vi "Set - Wash Sequence.vi"(8 "error in (no error)":errorcluster, 10 "Wash Sequence":T1[](array[typedef]), 11 "View Model":T2) -> (0 "error out":errorcluster, 3 "View Model":T2)   [LabVIEW 2017]
doc: "Set actual value of Wash Sequence to DVR."
uses:
  Controls/View Model.ctl
  Controls/Shared Model.ctl
  Error Handler/Controls/Error Model.ctl
  Error Handler/Controls/Error Data.ctl
  Error Handler/Controls/Error Level.ctl
  Configuration/Controls/Config Model.ctl
  Configuration/Controls/Config Record.ctl
  Configuration/Controls/Config Data.ctl
  Configuration/Controls/Config Command.ctl
  Controller/Controls/Controler Model.ctl
  Views/Vehicle Position View/Controls/Vehicle - Station Slider.ctl
  Controller/Controls/Controller - Wash Step.ctl
  Views/Entry Console View/Controls/Entry Console - Wash Steps.ctl
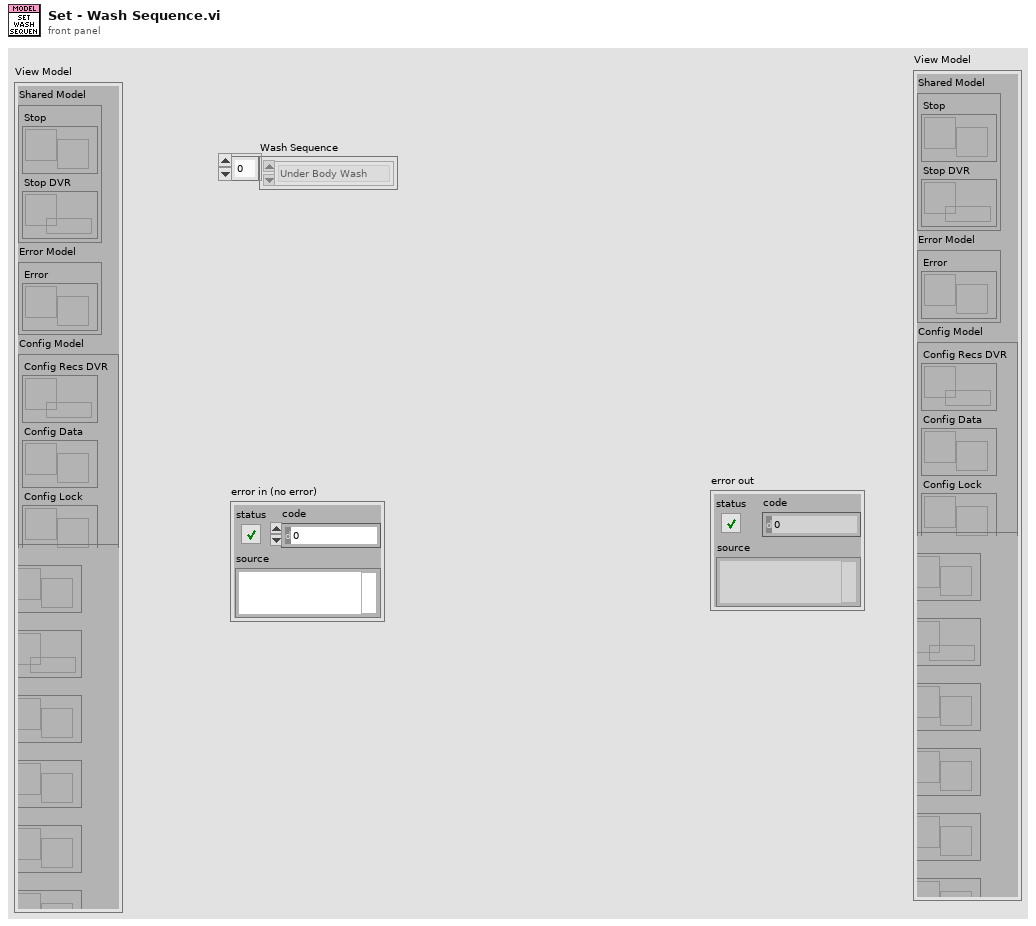
[diagram p1: front panel]
types:
  T1 = typedef "Controller - Wash Step.ctl" = enum16{"Under Body Wash", "Bug Remover", "Pre-Soak", "High Pressure Wash", "Low Pressure Wax", "Spot Free Rinse", "Tire Shine Foam", "Air Dry"}
  T2 = typedef "View Model.ctl" = cluster{"Shared Model":T3, "Error Model":T4, "Config Model":T5, "Controler Model":T6}
  T3 = typedef "Shared Model.ctl" = cluster{"Stop":refnum<user-event>, "Stop DVR":refnum<data-value>}
  T4 = typedef "Error Model.ctl" = cluster{"Error":refnum<user-event>}
  T5 = typedef "Config Model.ctl" = cluster{"Config Recs DVR":refnum<data-value>, "Config Data":refnum<user-event>, "Config Lock":refnum<user-event>, "Config Lock DVR":refnum<data-value>}
  T6 = typedef "Controler Model.ctl" = cluster{"Station":refnum<user-event>, "Wash Sequence":refnum<data-value>, "Wash Step Exec":refnum<user-event>, "Wash Step Start":refnum<user-event>, "Wash Step Complete":refnum<user-event>, "Wash Cycle Complete":refnum<user-event>, "Wash Cycle Start":refnum<user-event>}
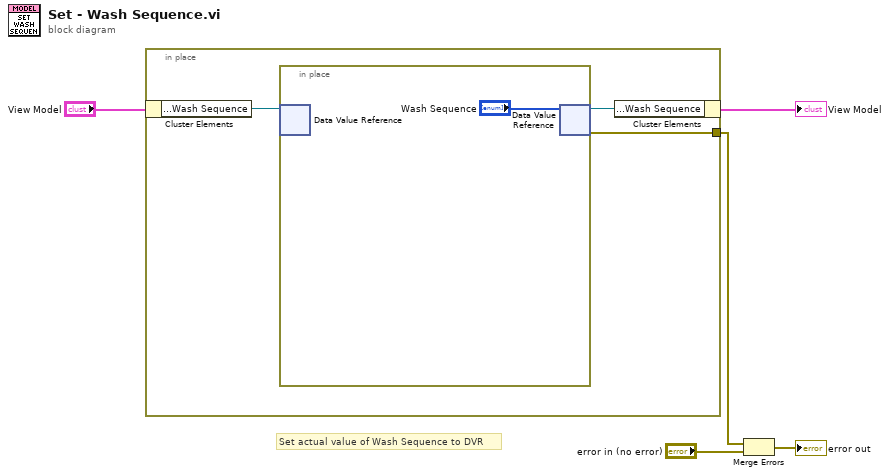
[diagram p0: block diagram]
diagram:
  # "Set actual value of Wash Sequence to DVR"
  n1 = in-place {
    in-place-border: [w6] -> w2
    n2 = in-place-cluster #1("View Model") -> ("Controler Model.Wash Sequence"=w8:refnum<data-value>)
    n3 = in-place {
      n4 = in-place-dvr #2(w8) -> ()  [unwired: 2 out]
      n5 = in-place-dvr #2("Wash Sequence") -> (w7:refnum<data-value>, w6:errorcluster)
    }
    n6 = in-place-cluster #1("Controler Model.Wash Sequence"=w7) -> (→"View Model":T2)
  }
  n7 = Merge Errors(w2, "error in (no error)") -> (→"error out":errorcluster)
